vi "uDAQsetDataRate.vi"(8 "error in (no error)":errorcluster, 10 "Menu Ring":T1(ring), 11 "connection ID":refnum<k5>) -> (0 "error out":errorcluster, 3 "connection ID out":refnum<k5>)   [LabVIEW 2017]
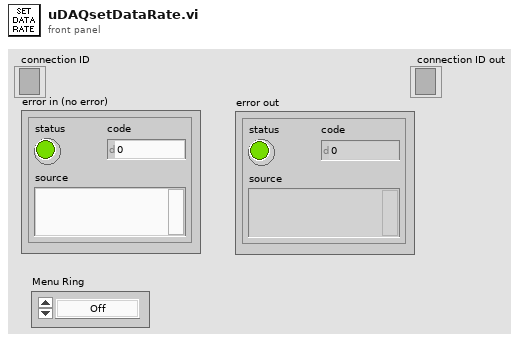
[diagram p1: front panel]
types:
  T1 = enum16{"Off", "1Hz", "5Hz", "10Hz", "20Hz", "25Hz", "50Hz", "100Hz", "150Hz", "200Hz", "225Hz", "312Hz", "400Hz", "500Hz", "625Hz", "1000Hz"}
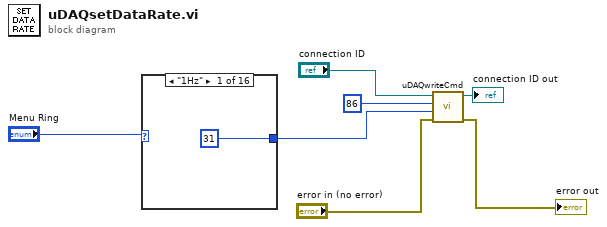
[diagram p0: block diagram]
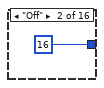
[diagram p2: hidden frame]
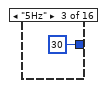
[diagram p3: hidden frame]
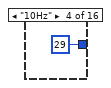
[diagram p4: hidden frame]
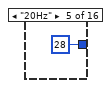
[diagram p5: hidden frame]
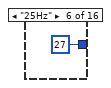
[diagram p6: hidden frame]
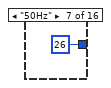
[diagram p7: hidden frame]
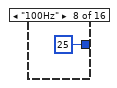
[diagram p8: hidden frame]
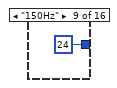
[diagram p9: hidden frame]
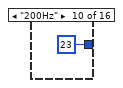
[diagram p10: hidden frame]
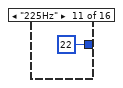
[diagram p11: hidden frame]
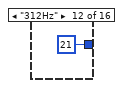
[diagram p12: hidden frame]
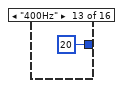
[diagram p13: hidden frame]
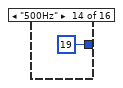
[diagram p14: hidden frame]
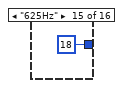
[diagram p15: hidden frame]
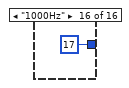
[diagram p16: hidden frame]
diagram:
  n1 = case shown="\"1Hz\"" "Menu Ring" {
    tunnel: [u8 31 ("ParamByte") u8 16 ("ParamByte") u8 30 ("ParamByte") u8 29 ("ParamByte") u8 28 ("ParamByte") u8 27 ("ParamByte") u8 26 ("ParamByte") u8 25 ("ParamByte") u8 24 ("ParamByte") u8 23 ("ParamByte") u8 22 ("ParamByte") u8 21 ("ParamByte") u8 20 ("ParamByte") u8 19 ("ParamByte") u8 18 ("ParamByte") u8 17 ("ParamByte")] -> w1
    frame "1Hz" {
    }
    frame "Off" {
    }
    frame "5Hz" {
    }
    frame "10Hz" {
    }
    frame "20Hz" {
    }
    frame "25Hz" {
    }
    frame "50Hz" {
    }
    frame "100Hz" {
    }
    frame "150Hz" {
    }
    frame "200Hz" {
    }
    frame "225Hz" {
    }
    frame "312Hz" {
    }
    frame "400Hz" {
    }
    frame "500Hz" {
    }
    frame "625Hz" {
    }
    frame "1000Hz" {
    }
  }
  n2 = call "uDAQwriteCmd.vi"("error in (no error)"="error in (no error)", "ParamByte"=w1, "CmdByte"=u8 86, "connection ID"="connection ID") -> ("error out"=→"error out":errorcluster, "connection ID out"=→"connection ID out":refnum<k5>)  [unwired: 6 in]
